vi "L09.vi"() -> ()   [LabVIEW 2012]
panel:
  out "B":i32
  out "Boolean":bool
  out "product":i32
  out "A":i32
  out "C":i32
  # "200375425"
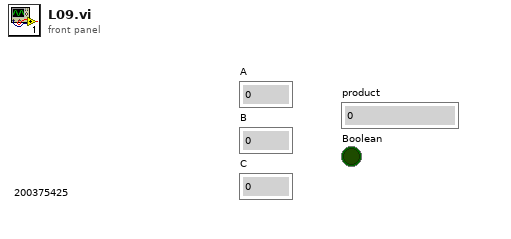
[diagram p1: front panel]
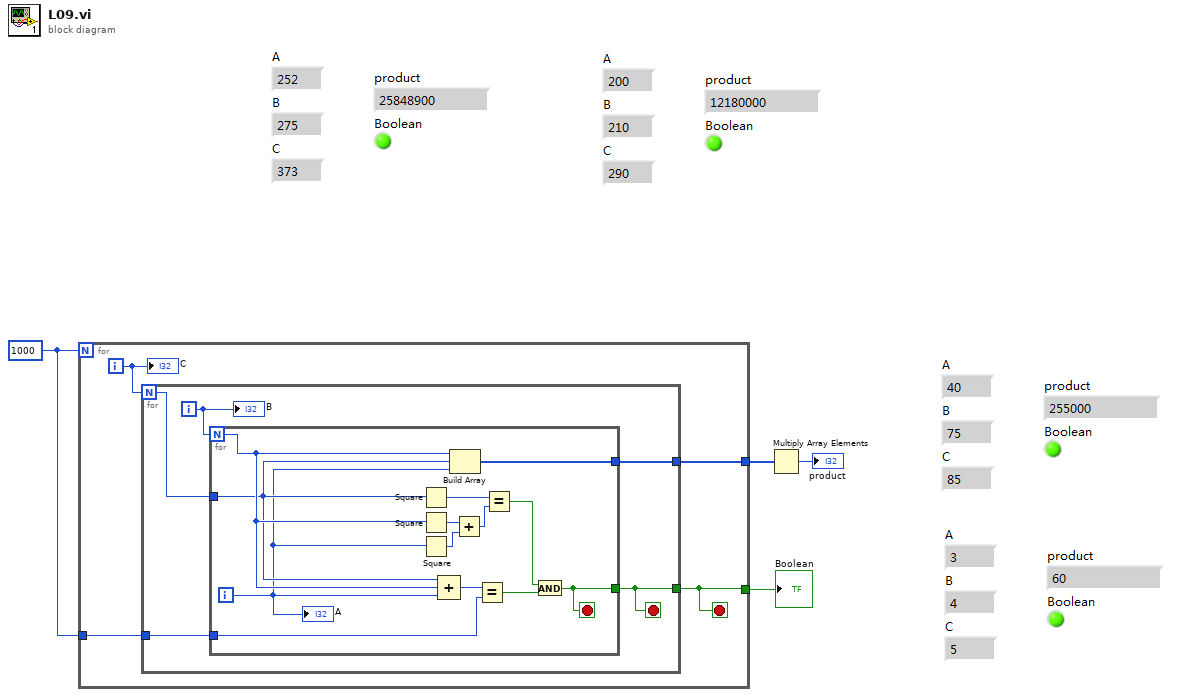
[diagram p0: block diagram]
diagram:
  w1 = 1000
  n1 = for {
    N: w1 -> [_]
    tunnel: [w7] -> w4
    tunnel: [w6] -> w2
    tunnel: w1 -> [w5]
    i -> [w8]
    stop <- w6 stop-if-true
    n2 = for {
      N: w8 -> [w13]
      tunnel: [w12] -> w6
      tunnel: [w11] -> w7
      tunnel: w5 -> [w9]
      i -> [w10]
      stop <- w12 stop-if-true
      n3 = for {
        N: w10 -> [w17]
        tunnel: w13 -> [w16]
        tunnel: [w19] -> w12
        tunnel: [w18] -> w11
        tunnel: w9 -> [w14]
        i -> [w15]
        stop <- w19 stop-if-true
        n4 = Square(x=w16) -> (x^2=w20:i32)
        n5 = Square(x=w17) -> (x^2=w21:i32)
        n6 = Square(x=w15) -> (x^2=w26:i32)
        n7 = Compound Arithmetic op=ADD(w16, w17, w15) -> (w24:i32)
        n8 = Build Array(w17, w16, w15) -> (w18:i32[])
        n9 = Add(x=w21, y=w26) -> (x+y=w25:i32)
        n10 = Equal?(x=w24, y=w14) -> (x = y?=w22:bool)
        n11 = Equal?(x=w20, y=w25) -> (x = y?=w23:bool)
        n12 = And(x=w23, y=w22) -> (x .and. y?=w19:bool)
        "A" <- w15
      }
      "B" <- w10
    }
    "C" <- w8
  }
  "Boolean" <- w2
  n13 = Multiply Array Elements(1:w4) -> (0:→"product":i32)
